vi "IncludedAngle.vi"(1 "CCW(T)":bool, 2 "upper limit":fxp<+,9,9>, 3 "lower limit":fxp<+,9,9>, 4 "angle":fxp<+/-,9,9>) -> (0 "s? t:f":bool)   [LabVIEW 2013]
doc: "Determine if an angle is included within the given angle range."
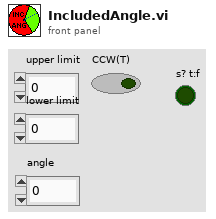
[diagram p1: front panel]
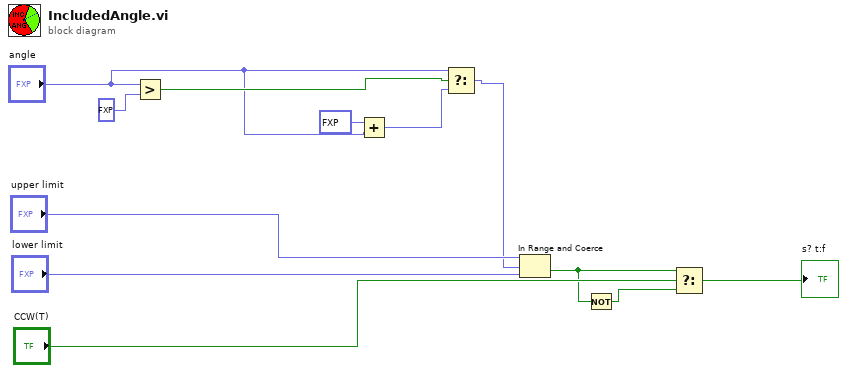
[diagram p0: block diagram]
diagram:
  n1 = Greater?(x="angle", y=fxp<+,9,9> 0.0) -> (0:w12:bool)
  n2 = Add(x=fxp<+,9,9> 360.0, y="angle") -> (x+y=w10:fxp<+/-,11,11>)
  n3 = Select(t="angle", s=w12, f=w10) -> (s? t:f=w7:fxp<+/-,11,11>)
  n4 = In Range and Coerce(upper limit="upper limit", x=w7, lower limit="lower limit") -> (In Range?=w2:bool)  [unwired: 1 out]
  n5 = Not(x=w2) -> (.not. x?=w1:bool)
  n6 = Select(t=w2, s="CCW(T)", f=w1) -> (s? t:f=→"s? t:f":bool)
